vi "Main.vi"(7 "sweep rate, /min":dbl=0.2, 8 "sweep to:":dbl=-0.5, 9 "sweep":T3(radio)=enum."time_sweep") -> ()   [LabVIEW 2017] (continued)
                          frame #12 {
                            # "check if voltage \non 2400 SouceMeter 3\nis to be measured"
                            n778 = property on="data" class="Arr (strict)"() -> ("Value"=w931:dbl[])  [unwired: 2 in, 2 out]
                            n779 = local read "2400 3 meas v"() -> (w930:bool)
                            n780 = case shown="True" w930 {
                              tunnel: w931 -> [w933 w944]
                              tunnel: [w933 w943] -> w932
                              frame False {
                                # "we are not measuring 2400 3, voltage (2400_3_v)"
                              }
                              frame True {
                                # "we are  measuring 2400 3, voltage (2400_3_v)"
                                n781 = local read "2400 3 addr"() -> (w938:u8)
                                n782 = Number To Decimal String(number=w938) -> (decimal integer string=w937:string)  [unwired: 1 in]
                                n783 = GPIB Write(0:w937, 1:":READ?") -> (6:w942:errorcluster)  [unwired: 3 in, 1 out]
                                n784 = GPIB Read(0:w937, 1:3200, 3:w942) -> (5:w935:string)  [unwired: 2 in, 2 out]
                                n785 = String Subset(string=w935, length (rest)=13) -> (substring=w934:string)  [unwired: 1 in]
                                n786 = Fract/Exp String To Number(string=w934) -> (number=w940:dbl)  [unwired: 3 in, 1 out]
                                n787 = Build Array (concatenate)(w944, w940) -> (w943:dbl[])
                              }
                            }
                            n788 = property on="data" class="Arr (strict)"("Value"=w932) -> ()  [unwired: 2 in, 2 out]
                          }
                          frame #13 {
                            # "check if current \non 2400 SouceMeter 3\nis to be measured"
                            n789 = property on="data" class="Arr (strict)"() -> ("Value"=w946:dbl[])  [unwired: 2 in, 2 out]
                            n790 = local read "2400 3 meas i"() -> (w945:bool)
                            n791 = case shown="True" w945 {
                              tunnel: w946 -> [w948 w960]
                              tunnel: [w948 w959] -> w947
                              frame False {
                                # "we are not measuring 2400 3, current (2400_3_i)"
                              }
                              frame True {
                                # "we are  measuring 2400 3, current (2400_3_i)"
                                n792 = local read "2400 3 addr"() -> (w954:u8)
                                n793 = Number To Decimal String(number=w954) -> (decimal integer string=w953:string)  [unwired: 1 in]
                                n794 = GPIB Write(0:w953, 1:":READ?") -> (6:w958:errorcluster)  [unwired: 3 in, 1 out]
                                n795 = GPIB Read(0:w953, 1:3200, 3:w958) -> (5:w951:string)  [unwired: 2 in, 2 out]
                                n796 = String Subset(string=w951, offset (0)=14, length (rest)=13) -> (substring=w950:string)
                                n797 = Fract/Exp String To Number(string=w950) -> (number=w956:dbl)  [unwired: 3 in, 1 out]
                                n798 = Build Array (concatenate)(w960, w956) -> (w959:dbl[])
                              }
                            }
                            n799 = property on="data" class="Arr (strict)"("Value"=w947) -> ()  [unwired: 2 in, 2 out]
                          }
                          frame #14 {
                            # "check if 1st channel \non Keithley 2182A 1\nis to be measured"
                            n800 = property on="data" class="Arr (strict)"() -> ("Value"=w962:dbl[])  [unwired: 2 in, 2 out]
                            n801 = local read "2182A 1 ch1"() -> (w961:bool)
                            n802 = case shown="True" w961 {
                              tunnel: w962 -> [w964 w973]
                              tunnel: [w964 w972] -> w963
                              frame False {
                                # "we are not measuring 2182A 1 channel 1 (2182A_1_ch1)"
                              }
                              frame True {
                                # "we are  measuring 2182A 1 channel 1 (2182A_1_ch1)"
                                n803 = local read "2182A 1 addr"() -> (w967:u8)
                                n804 = Number To Decimal String(number=w967) -> (decimal integer string=w966:string)  [unwired: 1 in]
                                n805 = GPIB Write(0:w966, 1:":SENSe:DATA:FRES?") -> (6:w971:errorcluster)  [unwired: 3 in, 1 out]
                                n806 = GPIB Read(0:w966, 1:200, 3:w971) -> (5:w965:string)  [unwired: 2 in, 2 out]
                                n807 = Fract/Exp String To Number(string=w965) -> (number=w969:dbl)  [unwired: 3 in, 1 out]
                                n808 = Build Array (concatenate)(w973, w969) -> (w972:dbl[])
                              }
                            }
                            n809 = property on="data" class="Arr (strict)"("Value"=w963) -> ()  [unwired: 2 in, 2 out]
                          }
                          frame #15 {
                            # "check if 2nd channel \non Keithley 2182A 1\nis to be measured"
                            n810 = property on="data" class="Arr (strict)"() -> ("Value"=w975:dbl[])  [unwired: 2 in, 2 out]
                            n811 = local read "2182A 1 ch2"() -> (w974:bool)
                            n812 = case shown="True" w974 {
                              tunnel: w975 -> [w977 w990]
                              tunnel: [w977 w989] -> w976
                              frame False {
                                # "we are not measuring 2182A 1 channel 2 (2182A_1_ch2)"
                              }
                              frame True {
                                # "switching to channel 2 and then\nback to channel 1"
                                # "we are  measuring 2182A 1 channel 2 (2182A_1_ch2)"
                                n813 = local read "2182A 1 addr"() -> (w984:u8)
                                n814 = Number To Decimal String(number=w984) -> (decimal integer string=w979:string)  [unwired: 1 in]
                                n815 = GPIB Write(0:w979, 1:":SENSe:CHAN 2") -> (6:w981:errorcluster)  [unwired: 3 in, 1 out]
                                n816 = GPIB Write(0:w979, 1:":SENSe:DATA:FRES?", 3:w981) -> (6:w988:errorcluster)  [unwired: 2 in, 1 out]
                                n817 = GPIB Read(0:w979, 1:200, 3:w988) -> (5:w983:string, 7:w980:errorcluster)  [unwired: 2 in, 1 out]
                                n818 = GPIB Write(0:w979, 1:":SENSe:CHAN 1", 3:w980) -> ()  [unwired: 2 in, 2 out]
                                n819 = Fract/Exp String To Number(string=w983) -> (number=w986:dbl)  [unwired: 3 in, 1 out]
                                n820 = Build Array (concatenate)(w990, w986) -> (w989:dbl[])
                              }
                            }
                            n821 = property on="data" class="Arr (strict)"("Value"=w976) -> ()  [unwired: 2 in, 2 out]
                          }
                          frame #16 {
                            # "check if 1st channel \non Keithley 2182A 2\nis to be measured"
                            n822 = property on="data" class="Arr (strict)"() -> ("Value"=w992:dbl[])  [unwired: 2 in, 2 out]
                            n823 = local read "2182A 2 ch1"() -> (w991:bool)
                            n824 = case shown="False" w991 {
                              tunnel: w992 -> [w994 w1003]
                              tunnel: [w994 w1002] -> w993
                              frame False {
                                # "we are not measuring 2182A 2 channel 1 (2182A_2_ch1)"
                              }
                              frame True {
                                # "we are  measuring 2182A 2 channel 1 (2182A_2_ch1)"
                                n825 = local read "2182A 2 addr"() -> (w997:u8)
                                n826 = Number To Decimal String(number=w997) -> (decimal integer string=w996:string)  [unwired: 1 in]
                                n827 = GPIB Write(0:w996, 1:":SENSe:DATA:FRES?") -> (6:w1001:errorcluster)  [unwired: 3 in, 1 out]
                                n828 = GPIB Read(0:w996, 1:200, 3:w1001) -> (5:w995:string)  [unwired: 2 in, 2 out]
                                n829 = Fract/Exp String To Number(string=w995) -> (number=w999:dbl)  [unwired: 3 in, 1 out]
                                n830 = Build Array (concatenate)(w1003, w999) -> (w1002:dbl[])
                              }
                            }
                            n831 = property on="data" class="Arr (strict)"("Value"=w993) -> ()  [unwired: 2 in, 2 out]
                          }
                          frame #17 {
                            # "check if 2nd channel \non Keithley 2182A 2\nis to be measured"
                            n832 = property on="data" class="Arr (strict)"() -> ("Value"=w1005:dbl[])  [unwired: 2 in, 2 out]
                            n833 = local read "2182A 2 ch2"() -> (w1004:bool)
                            n834 = case shown="True" w1004 {
                              tunnel: w1005 -> [w1007 w1020]
                              tunnel: [w1007 w1019] -> w1006
                              frame False {
                                # "we are not measuring 2182A 2 channel 2 (2182A_2_ch2)"
                              }
                              frame True {
                                # "switching to channel 2 and then\nback to channel 1"
                                # "we are  measuring 2182A 2 channel 2 (2182A_2_ch2)"
                                n835 = local read "2182A 2 addr"() -> (w1014:u8)
                                n836 = Number To Decimal String(number=w1014) -> (decimal integer string=w1009:string)  [unwired: 1 in]
                                n837 = GPIB Write(0:w1009, 1:":SENSe:CHAN 2") -> (6:w1011:errorcluster)  [unwired: 3 in, 1 out]
                                n838 = GPIB Write(0:w1009, 1:":SENSe:DATA:FRES?", 3:w1011) -> (6:w1018:errorcluster)  [unwired: 2 in, 1 out]
                                n839 = GPIB Read(0:w1009, 1:200, 3:w1018) -> (5:w1013:string, 7:w1010:errorcluster)  [unwired: 2 in, 1 out]
                                n840 = GPIB Write(0:w1009, 1:":SENSe:CHAN 1", 3:w1010) -> ()  [unwired: 2 in, 2 out]
                                n841 = Fract/Exp String To Number(string=w1013) -> (number=w1016:dbl)  [unwired: 3 in, 1 out]
                                n842 = Build Array (concatenate)(w1020, w1016) -> (w1019:dbl[])
                              }
                            }
                            n843 = property on="data" class="Arr (strict)"("Value"=w1006) -> ()  [unwired: 2 in, 2 out]
                          }
                          frame #18 {
                            # "check if 1st channel \non Keithley 2182A 3\nis to be measured"
                            n844 = property on="data" class="Arr (strict)"() -> ("Value"=w1022:dbl[])  [unwired: 2 in, 2 out]
                            n845 = local read "2182A 3 ch1"() -> (w1021:bool)
                            n846 = case shown="True" w1021 {
                              tunnel: w1022 -> [w1024 w1033]
                              tunnel: [w1024 w1032] -> w1023
                              frame False {
                                # "we are not measuring 2182A 3 channel 1 (2182A_3_ch1)"
                              }
                              frame True {
                                # "we are  measuring 2182A 3 channel 1 (2182A_3_ch1)"
                                n847 = local read "2182A 3 addr"() -> (w1027:u8)
                                n848 = Number To Decimal String(number=w1027) -> (decimal integer string=w1026:string)  [unwired: 1 in]
                                n849 = GPIB Write(0:w1026, 1:":SENSe:DATA:FRES?") -> (6:w1031:errorcluster)  [unwired: 3 in, 1 out]
                                n850 = GPIB Read(0:w1026, 1:200, 3:w1031) -> (5:w1025:string)  [unwired: 2 in, 2 out]
                                n851 = Fract/Exp String To Number(string=w1025) -> (number=w1029:dbl)  [unwired: 3 in, 1 out]
                                n852 = Build Array (concatenate)(w1033, w1029) -> (w1032:dbl[])
                              }
                            }
                            n853 = property on="data" class="Arr (strict)"("Value"=w1023) -> ()  [unwired: 2 in, 2 out]
                          }
                          frame #19 {
                            # "check if 2nd channel \non Keithley 2182A 3\nis to be measured"
                            n854 = property on="data" class="Arr (strict)"() -> ("Value"=w1035:dbl[])  [unwired: 2 in, 2 out]
                            n855 = local read "2182A 3 ch2"() -> (w1034:bool)
                            n856 = case shown="True" w1034 {
                              tunnel: w1035 -> [w1037 w1050]
                              tunnel: [w1037 w1049] -> w1036
                              frame False {
                                # "we are not measuring 2182A 3 channel 2 (2182A_3_ch2)"
                              }
                              frame True {
                                # "switching to channel 2 and then\nback to channel 1"
                                # "we are  measuring 2182A 3 channel 2 (2182A_3_ch2)"
                                n857 = local read "2182A 3 addr"() -> (w1044:u8)
                                n858 = Number To Decimal String(number=w1044) -> (decimal integer string=w1039:string)  [unwired: 1 in]
                                n859 = GPIB Write(0:w1039, 1:":SENSe:CHAN 2") -> (6:w1041:errorcluster)  [unwired: 3 in, 1 out]
                                n860 = GPIB Write(0:w1039, 1:":SENSe:DATA:FRES?", 3:w1041) -> (6:w1048:errorcluster)  [unwired: 2 in, 1 out]
                                n861 = GPIB Read(0:w1039, 1:200, 3:w1048) -> (5:w1043:string, 7:w1040:errorcluster)  [unwired: 2 in, 1 out]
                                n862 = GPIB Write(0:w1039, 1:":SENSe:CHAN 1", 3:w1040) -> ()  [unwired: 2 in, 2 out]
                                n863 = Fract/Exp String To Number(string=w1043) -> (number=w1046:dbl)  [unwired: 3 in, 1 out]
                                n864 = Build Array (concatenate)(w1050, w1046) -> (w1049:dbl[])
                              }
                            }
                            n865 = property on="data" class="Arr (strict)"("Value"=w1036) -> ()  [unwired: 2 in, 2 out]
                          }
                          frame #20 {
                            # "check if 1st channel \non Keithley 2182A 4\nis to be measured"
                            n866 = property on="data" class="Arr (strict)"() -> ("Value"=w1052:dbl[])  [unwired: 2 in, 2 out]
                            n867 = local read "2182A 4 ch1"() -> (w1051:bool)
                            n868 = case shown="True" w1051 {
                              tunnel: w1052 -> [w1054 w1063]
                              tunnel: [w1054 w1062] -> w1053
                              frame False {
                                # "we are not measuring 2182A 4 channel 1 (2182A_4_ch1)"
                              }
                              frame True {
                                # "we are  measuring 2182A 4 channel 1 (2182A_4_ch1)"
                                n869 = local read "2182A 4 addr"() -> (w1057:u8)
                                n870 = Number To Decimal String(number=w1057) -> (decimal integer string=w1056:string)  [unwired: 1 in]
                                n871 = GPIB Write(0:w1056, 1:":SENSe:DATA:FRES?") -> (6:w1061:errorcluster)  [unwired: 3 in, 1 out]
                                n872 = GPIB Read(0:w1056, 1:200, 3:w1061) -> (5:w1055:string)  [unwired: 2 in, 2 out]
                                n873 = Fract/Exp String To Number(string=w1055) -> (number=w1059:dbl)  [unwired: 3 in, 1 out]
                                n874 = Build Array (concatenate)(w1063, w1059) -> (w1062:dbl[])
                              }
                            }
                            n875 = property on="data" class="Arr (strict)"("Value"=w1053) -> ()  [unwired: 2 in, 2 out]
                          }
                          frame #21 {
                            # "check if 2nd channel \non Keithley 2182A 4\nis to be measured"
                            n876 = property on="data" class="Arr (strict)"() -> ("Value"=w1065:dbl[])  [unwired: 2 in, 2 out]
                            n877 = local read "2182A 4 ch2"() -> (w1064:bool)
                            n878 = case shown="False" w1064 {
                              tunnel: w1065 -> [w1067 w1080]
                              tunnel: [w1067 w1079] -> w1066
                              frame False {
                                # "we are not measuring 2182A 4 channel 2 (2182A_4_ch2)"
                              }
                              frame True {
                                # "switching to channel 2 and then\nback to channel 1"
                                # "we are  measuring 2182A 4 channel 2 (2182A_4_ch2)"
                                n879 = local read "2182A 4 addr"() -> (w1074:u8)
                                n880 = Number To Decimal String(number=w1074) -> (decimal integer string=w1069:string)  [unwired: 1 in]
                                n881 = GPIB Write(0:w1069, 1:":SENSe:CHAN 2") -> (6:w1071:errorcluster)  [unwired: 3 in, 1 out]
                                n882 = GPIB Write(0:w1069, 1:":SENSe:DATA:FRES?", 3:w1071) -> (6:w1078:errorcluster)  [unwired: 2 in, 1 out]
                                n883 = GPIB Read(0:w1069, 1:200, 3:w1078) -> (5:w1073:string, 7:w1070:errorcluster)  [unwired: 2 in, 1 out]
                                n884 = GPIB Write(0:w1069, 1:":SENSe:CHAN 1", 3:w1070) -> ()  [unwired: 2 in, 2 out]
                                n885 = Fract/Exp String To Number(string=w1073) -> (number=w1076:dbl)  [unwired: 3 in, 1 out]
                                n886 = Build Array (concatenate)(w1080, w1076) -> (w1079:dbl[])
                              }
                            }
                            n887 = property on="data" class="Arr (strict)"("Value"=w1066) -> ()  [unwired: 2 in, 2 out]
                          }
                          frame #22 {
                            # "check if voltage on\nKeithley 2636A smua\nis to be measured"
                            n888 = local read "2636A smua meas v"() -> (w1081:bool)
                            n889 = property on="data" class="Arr (strict)"() -> ("Value"=w1082:dbl[])  [unwired: 2 in, 2 out]
                            n890 = case shown="True" w1081 {
                              tunnel: w1082 -> [w1084 w1090]
                              tunnel: [w1084 w1089] -> w1083
                              frame False {
                                # "we are not measuring voltage on 2636A smua (2636A_smua_v)"
                              }
                              frame True {
                                # "we are  measuring voltage on 2636A smua (2636A_smua_v)"
                                n891 = local read "2336A addr"() -> (w1085:refnum<visa-resource-name>)
                                n892 = call "SinglePointMeasurement.vi"("Measure"=Measure."Voltage", "Channel"=Channel."a", "VISA resource name 2"=w1085) -> ("Measuremet"=w1087:dbl)  [unwired: 3 in, 4 out]
                                n893 = Build Array (concatenate)(w1090, w1087) -> (w1089:dbl[])
                              }
                            }
                            n894 = property on="data" class="Arr (strict)"("Value"=w1083) -> ()  [unwired: 2 in, 2 out]
                          }
                          frame #23 {
                            # "check if current on\nKeithley 2636A smua\nis to be measured"
                            n895 = local read "2636A smua meas i"() -> (w1091:bool)
                            n896 = property on="data" class="Arr (strict)"() -> ("Value"=w1092:dbl[])  [unwired: 2 in, 2 out]
                            n897 = case shown="True" w1091 {
                              tunnel: w1092 -> [w1094 w1097]
                              tunnel: [w1094 w1096] -> w1093
                              frame False {
                                # "we are not measuring current on 2636A smua (2636A_smua_i)"
                              }
                              frame True {
                                # "we are  measuring current on 2636A smua (2636A_smua_i)"
                                n898 = stacked-sequence {
                                tunnel: [_ w1106] -> w1095
                                frame #0 {
                                n899 = local read "auto\nrange A"() -> (w1101:bool)
                                n900 = local read "2336A addr"() -> (w1104:refnum<visa-resource-name>)
                                n901 = Select(t="smua.AUTORANGE_ON", s=w1101, f="smua.AUTORANGE_OFF") -> (s? t:f=w1099:string)
                                n902 = Concatenate Strings("smua.measure.autorangei = ", w1099) -> (w1098:string)
                                n903 = VISA Write(VISA resource name=w1104, write buffer=w1098) -> ()  [unwired: 1 in, 3 out]
                                }
                                frame #1 {
                                n904 = local read "2336A addr"() -> (w1108:refnum<visa-resource-name>)
                                n905 = call "SinglePointMeasurement.vi"("Measure"=Measure."Current", "Channel"=Channel."a", "VISA resource name 2"=w1108) -> ("Measuremet"=w1106:dbl)  [unwired: 3 in, 4 out]
                                }
                                }
                                n906 = Build Array (concatenate)(w1097, w1095) -> (w1096:dbl[])
                              }
                            }
                            n907 = property on="data" class="Arr (strict)"("Value"=w1093) -> ()  [unwired: 2 in, 2 out]
                          }
                          frame #24 {
                            # "check if voltage on\nKeithley 2636A smub\nis to be measured"
                            n908 = local read "2636A smub meas v"() -> (w1109:bool)
                            n909 = property on="data" class="Arr (strict)"() -> ("Value"=w1110:dbl[])  [unwired: 2 in, 2 out]
                            n910 = case shown="True" w1109 {
                              tunnel: w1110 -> [w1112 w1118]
                              tunnel: [w1112 w1117] -> w1111
                              frame False {
                                # "we are not measuring voltage on 2636A smub (2636A_smub_v)"
                              }
                              frame True {
                                # "we are  measuring voltage on 2636A smub (2636A_smub_v)"
                                n911 = local read "2336A addr"() -> (w1116:refnum<visa-resource-name>)
                                n912 = call "SinglePointMeasurement.vi"("Measure"=Measure."Voltage", "Channel"=Channel."b", "VISA resource name 2"=w1116) -> ("Measuremet"=w1114:dbl)  [unwired: 3 in, 4 out]
                                n913 = Build Array (concatenate)(w1118, w1114) -> (w1117:dbl[])
                              }
                            }
                            n914 = property on="data" class="Arr (strict)"("Value"=w1111) -> ()  [unwired: 2 in, 2 out]
                          }
                          frame #25 {
                            # "check if current on\nKeithley 2636A smub\nis to be measured"
                            n915 = local read "2636A smub meas i"() -> (w1119:bool)
                            n916 = property on="data" class="Arr (strict)"() -> ("Value"=w1120:dbl[])  [unwired: 2 in, 2 out]
                            n917 = case shown="True" w1119 {
                              tunnel: w1120 -> [w1122 w1125]
                              tunnel: [w1122 w1124] -> w1121
                              frame False {
                                # "we are not measuring current on 2636A smub (2636A_smub_i)"
                              }
                              frame True {
                                # "we are  measuring current on 2636A smub (2636A_smub_i)"
                                n918 = stacked-sequence {
                                tunnel: [_ w1134] -> w1123
                                frame #0 {
                                n919 = local read "auto\nrange B"() -> (w1129:bool)
                                n920 = local read "2336A addr"() -> (w1132:refnum<visa-resource-name>)
                                n921 = Select(t="smub.AUTORANGE_ON", s=w1129, f="smub.AUTORANGE_OFF") -> (s? t:f=w1127:string)
                                n922 = Concatenate Strings("smub.measure.autorangei = ", w1127) -> (w1126:string)
                                n923 = VISA Write(VISA resource name=w1132, write buffer=w1126) -> ()  [unwired: 1 in, 3 out]
                                }
                                frame #1 {
                                n924 = local read "2336A addr"() -> (w1136:refnum<visa-resource-name>)
                                n925 = call "SinglePointMeasurement.vi"("Measure"=Measure."Current", "Channel"=Channel."b", "VISA resource name 2"=w1136) -> ("Measuremet"=w1134:dbl)  [unwired: 3 in, 4 out]
                                }
                                }
                                n926 = Build Array (concatenate)(w1125, w1123) -> (w1124:dbl[])
                              }
                            }
                            n927 = property on="data" class="Arr (strict)"("Value"=w1121) -> ()  [unwired: 2 in, 2 out]
                          }
                          frame #26 {
                            # "check if time\nis to be measured"
                            n928 = property on="data" class="Arr (strict)"() -> ("Value"=w1138:dbl[])  [unwired: 2 in, 2 out]
                            n929 = local read "measure time"() -> (w1137:bool)
                            n930 = case shown="True" w1137 {
                              tunnel: w1138 -> [w1140 w1143]
                              tunnel: [w1140 w1142] -> w1139
                              frame False {
                                # "we are not measuring time"
                              }
                              frame True {
                                # "seconds from the beginning of month"
                                # "we are  measuring time"
                                n931 = Build Array (concatenate)(w1143, 0) -> (w1142:dbl[])
                              }
                            }
                            n932 = property on="data" class="Arr (strict)"("Value"=w1139) -> ()  [unwired: 2 in, 2 out]
                          }
                          frame #27 {
                            n933 = local read "iPS_MagnetField"() -> (w1145:bool)
                            n934 = property on="data" class="Arr (strict)"() -> ("Value"=w1146:dbl[])  [unwired: 2 in, 2 out]
                            n935 = case shown="True" w1145 {
                              tunnel: w1146 -> [_ w1155]
                              tunnel: [_ w1154] -> w1144
                              frame False {
                                # "we are not Measuring magnetic field on IPS120-0"
                              }
                              frame True {
                                w1149 = 1
                                # "Measure magnetic field on IPS120-0"
                                n936 = local read "IPS120-0 addr_sweep"() -> (w1151:u8)
                                n937 = Number To Decimal String(number=w1151) -> (decimal integer string=w1152:string)  [unwired: 1 in]
                                n938 = GPIB Write(0:w1152, 1:"R 7", 2:w1149) -> ()  [unwired: 2 in, 2 out]
                                n939 = GPIB Read(0:w1152, 1:200 ("byte count"), 2:w1149) -> (5:w1153:string)  [unwired: 2 in, 2 out]
                                n940 = Fract/Exp String To Number(string=w1153, offset=w1149) -> (number=w1147:dbl)  [unwired: 2 in, 1 out]
                                n941 = Build Array (concatenate)(w1155, w1147) -> (w1154:dbl[])
                              }
                            }
                            n942 = property on="data" class="Arr (strict)"("Value"=w1144) -> ()  [unwired: 2 in, 2 out]
                          }
                          frame #28 {
                            # "check if current \non 2461 SouceMeter\nis to be measured"
                            n943 = property on="data" class="Arr (strict)"() -> ("Value"=w1158:dbl[])  [unwired: 2 in, 2 out]
                            n944 = property on="iTC_Sample_T" class="Bool (strict)"() -> ("Value"=w1157:bool)  [unwired: 2 in, 2 out]
                            n945 = case shown="True" w1157 {
                              tunnel: w1158 -> [_ w1171]
                              tunnel: [_ w1170] -> w1156
                              frame False {
                                # "we are not measuring 2461, voltage (2461_meas_v)"
                              }
                              frame True {
                                w1160 = 1
                                # "temporarily ITC503S"
                                # "we are  measuring  Teslatron_iTC_Temp"
                                n946 = property on="iTC_503_addr_sweep" class="DigNum (strict)"() -> ("Value"=w1165:u8)  [unwired: 2 in, 2 out]
                                n947 = Number To Decimal String(number=w1165) -> (decimal integer string=w1166:string)  [unwired: 1 in]
                                n948 = GPIB Write(0:w1166, 1:"$C3", 2:1) -> (6:w1167:errorcluster)  [unwired: 2 in, 1 out]
                                n949 = GPIB Write(0:w1166, 1:"R3", 2:w1160, 3:w1167) -> (6:w1169:errorcluster)  [unwired: 1 in, 1 out]
                                n950 = GPIB Read(0:w1166, 1:200, 2:w1160, 3:w1169) -> (5:w1168:string)  [unwired: 1 in, 2 out]
                                n951 = Fract/Exp String To Number(string=w1168, offset=w1160) -> (number=w1159:dbl)  [unwired: 2 in, 1 out]
                                n952 = Build Array (concatenate)(w1171, w1159) -> (w1170:dbl[])
                              }
                            }
                            n953 = property on="data" class="Arr (strict)"("Value"=w1156) -> ()  [unwired: 2 in, 2 out]
                          }
                          frame #29 {
                            # "check if current \non 2461 SouceMeter\nis to be measured"
                            n954 = property on="CH_A" class="Bool (strict)"() -> ("Value"=w1172:bool)  [unwired: 2 in, 2 out]
                            n955 = property on="data" class="Arr (strict)"() -> ("Value"=w1173:dbl[])  [unwired: 2 in, 2 out]
                            n956 = case shown="True" w1172 {
                              tunnel: w1173 -> [w1175 w1188]
                              tunnel: [w1175 w1187] -> w1174
                              frame False {
                                # "we are not measuring 2461, voltage (2461_meas_v)"
                              }
                              frame True {
                                w1180 = 1
                                # "temporarily ITC503S"
                                # "we are  measuring  Teslatron_iTC_Temp"
                                n957 = property on="iTC_503_addr_sweep" class="DigNum (strict)"() -> ("Value"=w1182:u8)  [unwired: 2 in, 2 out]
                                n958 = Number To Decimal String(number=w1182) -> (decimal integer string=w1183:string)  [unwired: 1 in]
                                n959 = GPIB Write(0:w1183, 1:"$C3", 2:1) -> (6:w1184:errorcluster)  [unwired: 2 in, 1 out]
                                n960 = GPIB Write(0:w1183, 1:"R3", 2:w1180, 3:w1184) -> (6:w1186:errorcluster)  [unwired: 1 in, 1 out]
                                n961 = GPIB Read(0:w1183, 1:200, 2:w1180, 3:w1186) -> (5:w1185:string)  [unwired: 1 in, 2 out]
                                n962 = Fract/Exp String To Number(string=w1185, offset=w1180) -> (number=w1181:dbl)  [unwired: 2 in, 1 out]
                                n963 = Build Array (concatenate)(w1188, w1181) -> (w1187:dbl[])
                              }
                            }
                            n964 = property on="data" class="Arr (strict)"("Value"=w1174) -> ()  [unwired: 2 in, 2 out]
                          }
                          frame #30 {
                            # "check if current \non 2461 SouceMeter\nis to be measured"
                            n965 = property on="CH_B" class="Bool (strict)"() -> ("Value"=w1189:bool)  [unwired: 2 in, 2 out]
                            n966 = property on="data" class="Arr (strict)"() -> ("Value"=w1190:dbl[])  [unwired: 2 in, 2 out]
                            n967 = case shown="True" w1189 {
                              tunnel: w1190 -> [w1192 w1205]
                              tunnel: [w1192 w1204] -> w1191
                              frame False {
                                # "we are not measuring 2461, voltage (2461_meas_v)"
                              }
                              frame True {
                                w1196 = 1
                                # "temporarily ITC503S"
                                # "we are  measuring  Teslatron_iTC_Temp"
                                n968 = property on="iTC_503_addr_sweep" class="DigNum (strict)"() -> ("Value"=w1199:u8)  [unwired: 2 in, 2 out]
                                n969 = Number To Decimal String(number=w1199) -> (decimal integer string=w1200:string)  [unwired: 1 in]
                                n970 = GPIB Write(0:w1200, 1:"$C3", 2:1) -> (6:w1201:errorcluster)  [unwired: 2 in, 1 out]
                                n971 = GPIB Write(0:w1200, 1:"R2", 2:w1196, 3:w1201) -> (6:w1203:errorcluster)  [unwired: 1 in, 1 out]
                                n972 = GPIB Read(0:w1200, 1:200, 2:w1196, 3:w1203) -> (5:w1202:string)  [unwired: 1 in, 2 out]
                                n973 = Fract/Exp String To Number(string=w1202, offset=w1196) -> (number=w1193:dbl)  [unwired: 2 in, 1 out]
                                n974 = Build Array (concatenate)(w1205, w1193) -> (w1204:dbl[])
                              }
                            }
                            n975 = property on="data" class="Arr (strict)"("Value"=w1191) -> ()  [unwired: 2 in, 2 out]
                          }
                        }
                      }
                    }
                  }
                }
              }
            }
          }
          frame #3 {
            n976 = Enqueue Element(queue=w1206, element="Idle") -> ()  [unwired: 2 in, 3 out]
            n977 = Wait (ms)(milliseconds to wait="Refresh Time(ms)") -> ()  [unwired: 1 out]
          }
        }
      }
      frame "Start Sweep" {
        w1212 = dbl[][] []  # emty array for data
        # "0 = SR830_1_ip\n1 = SR830_1_oop\n2 = SR830_2_ip\n3 = SR830_2_oop\n4 = SR830_3_ip\n5 = SR830_3_oop\n6 = SR830_4_ip \n7 = SR830_4_oop \n8= 2400_1_v \n9 = 2400_1_i \n10 = 2400_2_v\n11 = 2400_2_i \n12 = 2400_3_v \n13 = 2400_3_i \n14 = 2182A_1_ch1 \n15 = 2182A_1_ch2 \n16 = 2182A_2_ch1 \n17 = 2182A_2_ch2\n18 = 2182A_3_ch1 \n19 = 2182A_3_ch2 \n20 = 2182A_4_ch1 \n21 = 2182A_4_ch2 \n22 = 2636A_smua_v \n23 = 2636A_smua_i \n24 = 2636A_smub_v \n25 = 2636A_smub_i \n26 = time\n27 = iPS_120\n28 = iTC _sample_T\n28 = iTC _CH_A\n29=iTC_CH_B\n31 = Step_Value"
        # "initial time in seconds\nfrom the beginning of month"
        n978 = call "timeInSeconds.vi"() -> ("Numeric"=w1213:dbl)  [unwired: 2 in, 1 out]
        n979 = stacked-sequence {
          tunnel: [_ _ w1755 _ _ _] -> w1209
          frame #0 {
            n980 = local read "2636A smua meas v"() -> (w1219:bool)
            n981 = local read "2636A smub meas v"() -> (w1217:bool)
            n982 = local read "2636A smub meas i"() -> (w1216:bool)
            n983 = local read "2636A smua meas i"() -> (w1218:bool)
            n984 = property on="sweep" class="RadioBtnsControl (strict)"() -> ("Value"=w1214:T3)  [unwired: 2 in, 2 out]
            n985 = Compound Arithmetic op=OR(w1219, w1218, w1217, w1216) -> (w1215:bool)
            n986 = case shown="\"2400_3\"" w1214 {
              frame "2400_1" {
                # "add label for the first column in the datafile"
                n987 = stacked-sequence {
                  frame #0 {
                    n988 = property on="data_caption" class="Str"("Value"="") -> ()  [unwired: 2 in, 2 out]
                    n989 = property on="Figure_axis" class="Arr (strict)"("Value"=string[] [] ("Figure_axis_string")) -> ()  [unwired: 2 in, 2 out]
                  }
                  frame #1 {
                    w1222 = "V_sweep_2400_1" ("V_sweep")
                    n990 = Concatenate Strings(w1222, "\t") -> (w1224:string)
                    n991 = Build Array(w1222) -> (w1223:string[])
                    n992 = property on="data_caption" class="Str"("Value"=w1224) -> ()  [unwired: 2 in, 2 out]
                    n993 = property on="Figure_axis" class="Arr (strict)"("Value"=w1223) -> ()  [unwired: 2 in, 2 out]
                  }
                }
              }
              frame "2400_2" {
                n994 = stacked-sequence {
                  frame #0 {
                    n995 = property on="data_caption" class="Str"("Value"="") -> ()  [unwired: 2 in, 2 out]
                    n996 = property on="Figure_axis" class="Arr (strict)"("Value"=string[] [] ("Figure_axis_string")) -> ()  [unwired: 2 in, 2 out]
                  }
                  frame #1 {
                    w1228 = "V_sweep_2400_2" ("V_sweep")
                    n997 = Build Array(w1228) -> (w1229:string[])
                    n998 = Concatenate Strings(w1228, "\t") -> (w1231:string)
                    n999 = property on="Figure_axis" class="Arr (strict)"("Value"=w1229) -> ()  [unwired: 2 in, 2 out]
                    n1000 = property on="data_caption" class="Str"("Value"=w1231) -> ()  [unwired: 2 in, 2 out]
                  }
                }
              }
              frame "2400_3" {
                n1001 = stacked-sequence {
                  frame #0 {
                    n1002 = property on="data_caption" class="Str"("Value"="") -> ()  [unwired: 2 in, 2 out]
                    n1003 = property on="Figure_axis" class="Arr (strict)"("Value"=string[] [] ("Figure_axis_string")) -> ()  [unwired: 2 in, 2 out]
                  }
                  frame #1 {
                    w1234 = "V_sweep_2400_3" ("V_sweep")
                    n1004 = Concatenate Strings(w1234, "\t") -> (w1237:string)
                    n1005 = Build Array(w1234) -> (w1235:string[])
                    n1006 = property on="data_caption" class="Str"("Value"=w1237) -> ()  [unwired: 2 in, 2 out]
                    n1007 = property on="Figure_axis" class="Arr (strict)"("Value"=w1235) -> ()  [unwired: 2 in, 2 out]
                  }
                }
              }
              frame "2636a_smua" {
                n1008 = stacked-sequence {
                  frame #0 {
                    n1009 = property on="data_caption" class="Str"("Value"="") -> ()  [unwired: 2 in, 2 out]
                    n1010 = property on="Figure_axis" class="Arr (strict)"("Value"=string[] [] ("Figure_axis_string")) -> ()  [unwired: 2 in, 2 out]
                  }
                  frame #1 {
                    w1240 = "V_sweep_2636a_smua" ("V_sweep")
                    n1011 = Concatenate Strings(w1240, "\t") -> (w1243:string)
                    n1012 = Build Array(w1240) -> (w1241:string[])
                    n1013 = property on="data_caption" class="Str"("Value"=w1243) -> ()  [unwired: 2 in, 2 out]
                    n1014 = property on="Figure_axis" class="Arr (strict)"("Value"=w1241) -> ()  [unwired: 2 in, 2 out]
                  }
                }
              }
              frame "2636a_smub" {
                n1015 = stacked-sequence {
                  frame #0 {
                    n1016 = property on="data_caption" class="Str"("Value"="") -> ()  [unwired: 2 in, 2 out]
                    n1017 = property on="Figure_axis" class="Arr (strict)"("Value"=string[] [] ("Figure_axis_string")) -> ()  [unwired: 2 in, 2 out]
                  }
                  frame #1 {
                    w1246 = "V_sweep_2636a_smub" ("V_sweep")
                    n1018 = Build Array(w1246) -> (w1247:string[])
                    n1019 = Concatenate Strings(w1246, "\t") -> (w1249:string)
                    n1020 = property on="Figure_axis" class="Arr (strict)"("Value"=w1247) -> ()  [unwired: 2 in, 2 out]
                    n1021 = property on="data_caption" class="Str"("Value"=w1249) -> ()  [unwired: 2 in, 2 out]
                  }
                }
              }
              frame "time_sweep", Default {
                n1022 = stacked-sequence {
                  frame #0 {
                    n1023 = property on="data_caption" class="Str"("Value"="") -> ()  [unwired: 2 in, 2 out]
                    n1024 = property on="Figure_axis" class="Arr (strict)"("Value"=string[] [] ("Figure_axis_string")) -> ()  [unwired: 2 in, 2 out]
                  }
                  frame #1 {
                    w1252 = "time_sweep" ("V_sweep")
                    n1025 = Build Array(w1252) -> (w1253:string[])
                    n1026 = Concatenate Strings(w1252, "\t") -> (w1254:string)
                    n1027 = property on="Figure_axis" class="Arr (strict)"("Value"=w1253) -> ()  [unwired: 2 in, 2 out]
                    n1028 = property on="data_caption" class="Str"("Value"=w1254) -> ()  [unwired: 2 in, 2 out]
                  }
                }
              }
              frame "iPS" {
                n1029 = stacked-sequence {
                  frame #0 {
                    n1030 = property on="data_caption" class="Str"("Value"="") -> ()  [unwired: 2 in, 2 out]
                    n1031 = property on="Figure_axis" class="Arr (strict)"("Value"=string[] [] ("Figure_axis_string")) -> ()  [unwired: 2 in, 2 out]
                  }
                  frame #1 {
                    w1258 = "Teslatron_iPS_OutputField" ("V_sweep")
                    n1032 = Build Array(w1258) -> (w1259:string[])
                    n1033 = Concatenate Strings(w1258, "\t") -> (w1261:string)
                    n1034 = property on="Figure_axis" class="Arr (strict)"("Value"=w1259) -> ()  [unwired: 2 in, 2 out]
                    n1035 = property on="data_caption" class="Str"("Value"=w1261) -> ()  [unwired: 2 in, 2 out]
                  }
                }
              }
              frame "iTC" {
                n1036 = stacked-sequence {
                  frame #0 {
                    n1037 = property on="data_caption" class="Str"("Value"="") -> ()  [unwired: 2 in, 2 out]
                    n1038 = property on="Figure_axis" class="Arr (strict)"("Value"=string[] ["", "SR830_1_ip", "SR830_1_oop", "SR830_2_ip", "SR830_2_oop", "2461_meas_v", "2461_meas_i", "2636A_smua_v", "2636A_smua_i", "formula"] ("Figure_axis")) -> ()  [unwired: 2 in, 2 out]
                  }
                  frame #1 {
                    w1266 = "Teslatron_iTC_Temp"
                    n1039 = Build Array(w1266) -> (w1265:string[])
                    n1040 = Concatenate Strings(w1266, "\t") -> (w1264:string)
                    n1041 = property on="data_caption" class="Str"("Value"=w1264) -> ()  [unwired: 2 in, 2 out]
                    n1042 = property on="Figure_axis" class="Arr (strict)"("Value"=w1265) -> ()  [unwired: 2 in, 2 out]
                  }
                }
              }
            }
            n1043 = case shown="True" w1215 {
              frame False {
              }
              frame True {
                # "opens session for 2636a system sourcemeter"
                n1044 = local read "2336A addr"() -> (w1268:refnum<visa-resource-name>)
                n1045 = VISA Open(VISA resource name=w1268) -> ()  [unwired: 4 in, 2 out]
              }
            }
          }
          frame #1 {
            # "0 = SR830_1_ip\n1 = SR830_1_oop\n2 = SR830_2_ip\n3 = SR830_2_oop\n4 = SR830_3_ip\n5 = SR830_3_oop\n6 = SR830_4_ip \n7 = SR830_4_oop \n8= 2400_1_v \n9 = 2400_1_i \n10 = 2400_2_v\n11 = 2400_2_i \n12 = 2400_3_v \n13 = 2400_3_i \n14 = 2182A_1_ch1 \n15 = 2182A_1_ch2 \n16 = 2182A_2_ch1 \n17 = 2182A_2_ch2\n18 = 2182A_3_ch1 \n19 = 2182A_3_ch2 \n20 = 2182A_4_ch1 \n21 = 2182A_4_ch2 \n22 = 2636A_smua_v \n23 = 2636A_smua_i \n24 = 2636A_smub_v \n25 = 2636A_smub_i \n26 = time\n27 = iPS_120\n28 = iTC _sample_T\n28 = iTC _CH_A\n29=iTC_CH_B\n31 = Step_Value"
            # "this part constructs the first (text) line for the data file with names of all measured variables,\nalso constructs a text array contaning names of all measured variable for the \"ring\" (so parameter can be selected and plotted)"
            n1046 = stacked-sequence {
              tunnel: [w1269 _ _ _ _ _ _ _ _ _ _ _ _ _ _ _ _ _ _ _ _ _ _ _ _ _ _ _ _ _ _ _] -> _
              frame #0 {
                # "SR830 1 in phase (SR830_1_ip)"
                n1047 = local read "SR830 1 ip"() -> (w1274:bool)
                n1048 = property on="Figure_axis" class="Arr (strict)"() -> ("Value"=w1271:string[])  [unwired: 2 in, 2 out]
                n1049 = property on="data_caption" class="Str"() -> ("Value"=w1273:string)  [unwired: 2 in, 2 out]
                n1050 = case shown="True" w1274 {
                  tunnel: w1273 -> [w1276 w1282]
                  tunnel: [w1276 w1281] -> w1272
                  tunnel: w1271 -> [w1275 w1279]
                  tunnel: [w1275 w1277] -> w1270
                  frame False {
                    # "not measure SR830 1 in phase signal (SR830_1_ip)"
                  }
                  frame True {
                    w1278 = "SR830_1_ip"
                    # "measure SR830 1 in phase signal (SR830_1_ip)"
                    n1051 = local read "SR830 1 addr"() -> (w1283:u8)
                    n1052 = Number To Decimal String(number=w1283) -> (decimal integer string=w1284:string)  [unwired: 1 in]
                    n1053 = GPIB Clear(3:w1284) -> ()  [unwired: 1 in, 2 out]
                    n1054 = Build Array (concatenate)(w1279, w1278) -> (w1277:string[])
                    n1055 = Concatenate Strings(w1282, w1278, "\t") -> (w1281:string)
                  }
                }
                n1056 = property on="Figure_axis" class="Arr (strict)"("Value"=w1270) -> ()  [unwired: 2 in, 2 out]
                n1057 = property on="data_caption" class="Str"("Value"=w1272) -> (error out=w1269:errorcluster)  [unwired: 2 in, 1 out]
              }
              frame #1 {
                # "SR830 1 out of phase (SR830_1_oop)"
                n1058 = local read "SR830 1 oop"() -> (w1289:bool)
                n1059 = property on="Figure_axis" class="Arr (strict)"() -> ("Value"=w1286:string[])  [unwired: 2 in, 2 out]
                n1060 = property on="data_caption" class="Str"() -> ("Value"=w1288:string)  [unwired: 2 in, 2 out]
                n1061 = case shown="False" w1289 {
                  tunnel: w1288 -> [w1291 w1297]
                  tunnel: [w1291 w1296] -> w1287
                  tunnel: w1286 -> [w1290 w1294]
                  tunnel: [w1290 w1292] -> w1285
                  frame False {
                    # "not measure SR830 1 out of phase signal (SR830_1_oop)"
                  }
                  frame True {
                    w1293 = "SR830_1_oop"
                    # "measure SR830 1 out of phase signal (SR830_1_oop)"
                    n1062 = local read "SR830 1 addr"() -> (w1298:u8)
                    n1063 = Number To Decimal String(number=w1298) -> (decimal integer string=w1299:string)  [unwired: 1 in]
                    n1064 = GPIB Clear(3:w1299) -> ()  [unwired: 1 in, 2 out]
                    n1065 = Build Array (concatenate)(w1294, w1293) -> (w1292:string[])
                    n1066 = Concatenate Strings(w1297, w1293, "\t") -> (w1296:string)
                  }
                }
                n1067 = property on="Figure_axis" class="Arr (strict)"("Value"=w1285) -> ()  [unwired: 2 in, 2 out]
                n1068 = property on="data_caption" class="Str"("Value"=w1287) -> ()  [unwired: 2 in, 2 out]
              }
              frame #2 {
                # "SR830 2 in phase (SR830_2_ip)"
                n1069 = local read "SR830 2 ip"() -> (w1304:bool)
                n1070 = property on="Figure_axis" class="Arr (strict)"() -> ("Value"=w1301:string[])  [unwired: 2 in, 2 out]
                n1071 = property on="data_caption" class="Str"() -> ("Value"=w1303:string)  [unwired: 2 in, 2 out]
                n1072 = case shown="False" w1304 {
                  tunnel: w1303 -> [w1306 w1312]
                  tunnel: [w1306 w1311] -> w1302
                  tunnel: w1301 -> [w1305 w1309]
                  tunnel: [w1305 w1307] -> w1300
                  frame False {
                    # "not measure SR830 2 in phase signal (SR830_2_ip)"
                  }
                  frame True {
                    w1308 = "SR830_2_ip"
                    # "measure SR830 2 in phase signal (SR830_2_ip)"
                    n1073 = local read "SR830 2 addr"() -> (w1313:u8)
                    n1074 = Number To Decimal String(number=w1313) -> (decimal integer string=w1314:string)  [unwired: 1 in]
                    n1075 = GPIB Clear(3:w1314) -> ()  [unwired: 1 in, 2 out]
                    n1076 = Build Array (concatenate)(w1309, w1308) -> (w1307:string[])
                    n1077 = Concatenate Strings(w1312, w1308, "\t") -> (w1311:string)
                  }
                }
                n1078 = property on="Figure_axis" class="Arr (strict)"("Value"=w1300) -> ()  [unwired: 2 in, 2 out]
                n1079 = property on="data_caption" class="Str"("Value"=w1302) -> ()  [unwired: 2 in, 2 out]
              }
              frame #3 {
                # "SR830 2 out of phase (SR830_2_oop)"
                n1080 = local read "SR830 2 oop"() -> (w1319:bool)
                n1081 = property on="Figure_axis" class="Arr (strict)"() -> ("Value"=w1316:string[])  [unwired: 2 in, 2 out]
                n1082 = property on="data_caption" class="Str"() -> ("Value"=w1318:string)  [unwired: 2 in, 2 out]
                n1083 = case shown="False" w1319 {
                  tunnel: w1318 -> [w1321 w1327]
                  tunnel: [w1321 w1326] -> w1317
                  tunnel: w1316 -> [w1320 w1324]
                  tunnel: [w1320 w1322] -> w1315
                  frame False {
                    # "not measure SR830 2 out of phase signal (SR830_2_oop)"
                  }
                  frame True {
                    w1323 = "SR830_2_oop"
                    # "measure SR830 2 out of phase signal (SR830_2_oop)"
                    n1084 = local read "SR830 2 addr"() -> (w1328:u8)
                    n1085 = Number To Decimal String(number=w1328) -> (decimal integer string=w1329:string)  [unwired: 1 in]
                    n1086 = GPIB Clear(3:w1329) -> ()  [unwired: 1 in, 2 out]
                    n1087 = Build Array (concatenate)(w1324, w1323) -> (w1322:string[])
                    n1088 = Concatenate Strings(w1327, w1323, "\t") -> (w1326:string)
                  }
                }
                n1089 = property on="Figure_axis" class="Arr (strict)"("Value"=w1315) -> ()  [unwired: 2 in, 2 out]
                n1090 = property on="data_caption" class="Str"("Value"=w1317) -> ()  [unwired: 2 in, 2 out]
              }
              frame #4 {
                # "SR830 3 in phase (SR830_3_ip)"
                n1091 = local read "SR830 3 ip"() -> (w1334:bool)
                n1092 = property on="Figure_axis" class="Arr (strict)"() -> ("Value"=w1331:string[])  [unwired: 2 in, 2 out]
                n1093 = property on="data_caption" class="Str"() -> ("Value"=w1333:string)  [unwired: 2 in, 2 out]
                n1094 = case shown="False" w1334 {
                  tunnel: w1333 -> [w1336 w1342]
                  tunnel: [w1336 w1341] -> w1332
                  tunnel: w1331 -> [w1335 w1339]
                  tunnel: [w1335 w1337] -> w1330
                  frame False {
                    # "not measure SR830 3 in phase signal (SR830_3_ip)"
                  }
                  frame True {
                    w1338 = "SR830_3_ip"
                    # "measure SR830 3 in phase signal (SR830_3_ip)"
                    n1095 = local read "SR830 3 addr"() -> (w1343:u8)
                    n1096 = Number To Decimal String(number=w1343) -> (decimal integer string=w1344:string)  [unwired: 1 in]
                    n1097 = GPIB Clear(3:w1344) -> ()  [unwired: 1 in, 2 out]
                    n1098 = Build Array (concatenate)(w1339, w1338) -> (w1337:string[])
                    n1099 = Concatenate Strings(w1342, w1338, "\t") -> (w1341:string)
                  }
                }
                n1100 = property on="Figure_axis" class="Arr (strict)"("Value"=w1330) -> ()  [unwired: 2 in, 2 out]
                n1101 = property on="data_caption" class="Str"("Value"=w1332) -> ()  [unwired: 2 in, 2 out]
              }
              frame #5 {
                # "SR830 3 out of phase (SR830_3_oop)"
                n1102 = local read "SR830 3 oop"() -> (w1349:bool)
                n1103 = property on="Figure_axis" class="Arr (strict)"() -> ("Value"=w1346:string[])  [unwired: 2 in, 2 out]
                n1104 = property on="data_caption" class="Str"() -> ("Value"=w1348:string)  [unwired: 2 in, 2 out]
                n1105 = case shown="False" w1349 {
                  tunnel: w1348 -> [w1351 w1357]
                  tunnel: [w1351 w1356] -> w1347
                  tunnel: w1346 -> [w1350 w1354]
                  tunnel: [w1350 w1352] -> w1345
                  frame False {
                    # "not measure SR830 3 out of phase signal (SR830_3_oop)"
                  }
                  frame True {
                    w1353 = "SR830_3_oop"
                    # "measure SR830 3 out phase signal (SR830_3_oop)"
                    n1106 = local read "SR830 3 addr"() -> (w1358:u8)
                    n1107 = Number To Decimal String(number=w1358) -> (decimal integer string=w1359:string)  [unwired: 1 in]
                    n1108 = GPIB Clear(3:w1359) -> ()  [unwired: 1 in, 2 out]
                    n1109 = Build Array (concatenate)(w1354, w1353) -> (w1352:string[])
                    n1110 = Concatenate Strings(w1357, w1353, "\t") -> (w1356:string)
                  }
                }
                n1111 = property on="Figure_axis" class="Arr (strict)"("Value"=w1345) -> ()  [unwired: 2 in, 2 out]
                n1112 = property on="data_caption" class="Str"("Value"=w1347) -> ()  [unwired: 2 in, 2 out]
              }
              frame #6 {
                # "SR830 4 in phase (SR830_4_ip)"
                n1113 = local read "SR830 4 ip"() -> (w1364:bool)
                n1114 = property on="Figure_axis" class="Arr (strict)"() -> ("Value"=w1361:string[])  [unwired: 2 in, 2 out]
                n1115 = property on="data_caption" class="Str"() -> ("Value"=w1363:string)  [unwired: 2 in, 2 out]
                n1116 = case shown="False" w1364 {
                  tunnel: w1363 -> [w1366 w1372]
                  tunnel: [w1366 w1371] -> w1362
                  tunnel: w1361 -> [w1365 w1369]
                  tunnel: [w1365 w1367] -> w1360
                  frame False {
                    # "not measure SR830 4 in phase signal (SR830_4_ip)"
                  }
                  frame True {
                    w1368 = "SR830_4_ip"
                    # "measure SR830 4 in phase signal (SR830_4_ip)"
                    n1117 = local read "SR830 4 addr"() -> (w1373:u8)
                    n1118 = Number To Decimal String(number=w1373) -> (decimal integer string=w1374:string)  [unwired: 1 in]
                    n1119 = GPIB Clear(3:w1374) -> ()  [unwired: 1 in, 2 out]
                    n1120 = Build Array (concatenate)(w1369, w1368) -> (w1367:string[])
                    n1121 = Concatenate Strings(w1372, w1368, "\t") -> (w1371:string)
                  }
                }
                n1122 = property on="Figure_axis" class="Arr (strict)"("Value"=w1360) -> ()  [unwired: 2 in, 2 out]
                n1123 = property on="data_caption" class="Str"("Value"=w1362) -> ()  [unwired: 2 in, 2 out]
              }
              frame #7 {
                # "SR830 4 out of phase (SR830_4_oop)"
                n1124 = local read "SR830 4 oop"() -> (w1379:bool)
                n1125 = property on="Figure_axis" class="Arr (strict)"() -> ("Value"=w1376:string[])  [unwired: 2 in, 2 out]
                n1126 = property on="data_caption" class="Str"() -> ("Value"=w1378:string)  [unwired: 2 in, 2 out]
                n1127 = case shown="False" w1379 {
                  tunnel: w1378 -> [w1381 w1387]
                  tunnel: [w1381 w1386] -> w1377
                  tunnel: w1376 -> [w1380 w1384]
                  tunnel: [w1380 w1382] -> w1375
                  frame False {
                    # "not measure SR830 4 out of phase signal (SR830_4_oop)"
                  }
                  frame True {
                    w1383 = "SR830_4_oop"
                    # "measure SR830 4 out of phase signal (SR830_4_oop)"
                    n1128 = local read "SR830 4 addr"() -> (w1388:u8)
                    n1129 = Number To Decimal String(number=w1388) -> (decimal integer string=w1389:string)  [unwired: 1 in]
                    n1130 = GPIB Clear(3:w1389) -> ()  [unwired: 1 in, 2 out]
                    n1131 = Build Array (concatenate)(w1384, w1383) -> (w1382:string[])
                    n1132 = Concatenate Strings(w1387, w1383, "\t") -> (w1386:string)
                  }
                }
                n1133 = property on="Figure_axis" class="Arr (strict)"("Value"=w1375) -> ()  [unwired: 2 in, 2 out]
                n1134 = property on="data_caption" class="Str"("Value"=w1377) -> ()  [unwired: 2 in, 2 out]
              }
              frame #8 {
                # "2400 1 voltage measure (2400_1_v)"
                n1135 = local read "2400 1 meas v"() -> (w1394:bool)
                n1136 = property on="Figure_axis" class="Arr (strict)"() -> ("Value"=w1391:string[])  [unwired: 2 in, 2 out]
                n1137 = property on="data_caption" class="Str"() -> ("Value"=w1393:string)  [unwired: 2 in, 2 out]
                n1138 = case shown="False" w1394 {
                  tunnel: w1393 -> [w1396 w1402]
                  tunnel: [w1396 w1401] -> w1392
                  tunnel: w1391 -> [w1395 w1399]
                  tunnel: [w1395 w1397] -> w1390
                  frame False {
                    # "not measure 2400 1 voltage (2400_1_v)"
                  }
                  frame True {
                    w1398 = "2400_1_v"
                    # "measure 2400 1 voltage (2400_1_v)"
                    n1139 = local read "2400 1 addr"() -> (w1403:u8)
                    n1140 = Number To Decimal String(number=w1403) -> (decimal integer string=w1404:string)  [unwired: 1 in]
                    n1141 = GPIB Clear(3:w1404) -> ()  [unwired: 1 in, 2 out]
                    n1142 = Build Array (concatenate)(w1399, w1398) -> (w1397:string[])
                    n1143 = Concatenate Strings(w1402, w1398, "\t") -> (w1401:string)
                  }
                }
                n1144 = property on="Figure_axis" class="Arr (strict)"("Value"=w1390) -> ()  [unwired: 2 in, 2 out]
                n1145 = property on="data_caption" class="Str"("Value"=w1392) -> ()  [unwired: 2 in, 2 out]
              }
              frame #9 {
                # "2400 1 current measure (2400_1_i)"
                n1146 = local read "2400 1 meas i"() -> (w1409:bool)
                n1147 = property on="Figure_axis" class="Arr (strict)"() -> ("Value"=w1406:string[])  [unwired: 2 in, 2 out]
                n1148 = property on="data_caption" class="Str"() -> ("Value"=w1408:string)  [unwired: 2 in, 2 out]
                n1149 = case shown="False" w1409 {
                  tunnel: w1408 -> [w1411 w1417]
                  tunnel: [w1411 w1416] -> w1407
                  tunnel: w1406 -> [w1410 w1414]
                  tunnel: [w1410 w1412] -> w1405
                  frame False {
                    # "not measure 2400 1 current (2400_1_i)"
                  }
                  frame True {
                    w1413 = "2400_1_i"
                    # "measure 2400 1 current (2400_1_i)"
                    n1150 = local read "2400 1 addr"() -> (w1418:u8)
                    n1151 = Number To Decimal String(number=w1418) -> (decimal integer string=w1419:string)  [unwired: 1 in]
                    n1152 = GPIB Clear(3:w1419) -> ()  [unwired: 1 in, 2 out]
                    n1153 = Build Array (concatenate)(w1414, w1413) -> (w1412:string[])
                    n1154 = Concatenate Strings(w1417, w1413, "\t") -> (w1416:string)
                  }
                }
                n1155 = property on="Figure_axis" class="Arr (strict)"("Value"=w1405) -> ()  [unwired: 2 in, 2 out]
                n1156 = property on="data_caption" class="Str"("Value"=w1407) -> ()  [unwired: 2 in, 2 out]
              }
              frame #10 {
                # "2400 2 voltage measure (2400_2_v)"
                n1157 = local read "2400 2 meas v"() -> (w1424:bool)
                n1158 = property on="Figure_axis" class="Arr (strict)"() -> ("Value"=w1421:string[])  [unwired: 2 in, 2 out]
                n1159 = property on="data_caption" class="Str"() -> ("Value"=w1423:string)  [unwired: 2 in, 2 out]
                n1160 = case shown="False" w1424 {
                  tunnel: w1423 -> [w1426 w1432]
                  tunnel: [w1426 w1431] -> w1422
                  tunnel: w1421 -> [w1425 w1429]
                  tunnel: [w1425 w1427] -> w1420
                  frame False {
                    # "not measure 2400 2 voltage (2400_2_v)"
                  }
                  frame True {
                    w1428 = "2400_2_v"
                    # "measure 2400 2 voltage (2400_2_v)"
                    n1161 = local read "2400 2 addr"() -> (w1433:u8)
                    n1162 = Number To Decimal String(number=w1433) -> (decimal integer string=w1434:string)  [unwired: 1 in]
                    n1163 = GPIB Clear(3:w1434) -> ()  [unwired: 1 in, 2 out]
                    n1164 = Build Array (concatenate)(w1429, w1428) -> (w1427:string[])
                    n1165 = Concatenate Strings(w1432, w1428, "\t") -> (w1431:string)
                  }
                }
                n1166 = property on="Figure_axis" class="Arr (strict)"("Value"=w1420) -> ()  [unwired: 2 in, 2 out]
                n1167 = property on="data_caption" class="Str"("Value"=w1422) -> ()  [unwired: 2 in, 2 out]
              }
              frame #11 {
                # "2400 2 current measure (2400_2_i)"
                n1168 = local read "2400 2 meas i"() -> (w1439:bool)
                n1169 = property on="Figure_axis" class="Arr (strict)"() -> ("Value"=w1436:string[])  [unwired: 2 in, 2 out]
                n1170 = property on="data_caption" class="Str"() -> ("Value"=w1438:string)  [unwired: 2 in, 2 out]
                n1171 = case shown="False" w1439 {
                  tunnel: w1438 -> [w1441 w1447]
                  tunnel: [w1441 w1446] -> w1437
                  tunnel: w1436 -> [w1440 w1444]
                  tunnel: [w1440 w1442] -> w1435
                  frame False {
                    # "not measure 2400 2 current (2400_2_i)"
                  }
                  frame True {
                    w1443 = "2400_2_i"
                    # "measure 2400 2 current (2400_2_i)"
                    n1172 = local read "2400 2 addr"() -> (w1448:u8)
                    n1173 = Number To Decimal String(number=w1448) -> (decimal integer string=w1449:string)  [unwired: 1 in]
                    n1174 = GPIB Clear(3:w1449) -> ()  [unwired: 1 in, 2 out]
                    n1175 = Build Array (concatenate)(w1444, w1443) -> (w1442:string[])
                    n1176 = Concatenate Strings(w1447, w1443, "\t") -> (w1446:string)
                  }
                }
                n1177 = property on="Figure_axis" class="Arr (strict)"("Value"=w1435) -> ()  [unwired: 2 in, 2 out]
                n1178 = property on="data_caption" class="Str"("Value"=w1437) -> ()  [unwired: 2 in, 2 out]
              }
              frame #12 {
                # "2400 3 voltage measure (2400_3_v)"
                n1179 = local read "2400 3 meas v"() -> (w1454:bool)
                n1180 = property on="Figure_axis" class="Arr (strict)"() -> ("Value"=w1451:string[])  [unwired: 2 in, 2 out]
                n1181 = property on="data_caption" class="Str"() -> ("Value"=w1453:string)  [unwired: 2 in, 2 out]
                n1182 = case shown="False" w1454 {
                  tunnel: w1453 -> [w1456 w1462]
                  tunnel: [w1456 w1461] -> w1452
                  tunnel: w1451 -> [w1455 w1459]
                  tunnel: [w1455 w1457] -> w1450
                  frame False {
                    # "not measure 2400 3 voltage (2400_3_v)"
                  }
                  frame True {
                    w1458 = "2400_3_v"
                    # "measure 2400 3 voltage (2400_3_v)"
                    n1183 = local read "2400 3 addr"() -> (w1463:u8)
                    n1184 = Number To Decimal String(number=w1463) -> (decimal integer string=w1464:string)  [unwired: 1 in]
                    n1185 = GPIB Clear(3:w1464) -> ()  [unwired: 1 in, 2 out]
                    n1186 = Build Array (concatenate)(w1459, w1458) -> (w1457:string[])
                    n1187 = Concatenate Strings(w1462, w1458, "\t") -> (w1461:string)
                  }
                }
                n1188 = property on="Figure_axis" class="Arr (strict)"("Value"=w1450) -> ()  [unwired: 2 in, 2 out]
                n1189 = property on="data_caption" class="Str"("Value"=w1452) -> ()  [unwired: 2 in, 2 out]
              }
              frame #13 {
                # "2400 3 current measure (2400_3_i)"
                n1190 = local read "2400 3 meas i"() -> (w1469:bool)
                n1191 = property on="Figure_axis" class="Arr (strict)"() -> ("Value"=w1466:string[])  [unwired: 2 in, 2 out]
                n1192 = property on="data_caption" class="Str"() -> ("Value"=w1468:string)  [unwired: 2 in, 2 out]
                n1193 = case shown="True" w1469 {
                  tunnel: w1468 -> [w1471 w1477]
                  tunnel: [w1471 w1476] -> w1467
                  tunnel: w1466 -> [w1470 w1474]
                  tunnel: [w1470 w1472] -> w1465
                  frame False {
                    # "not measure 2400 3 current (2400_3_i)"
                  }
                  frame True {
                    w1473 = "2400_3_i"
                    # "measure 2400 3 current (2400_3_i)"
                    n1194 = local read "2400 3 addr"() -> (w1478:u8)
                    n1195 = Number To Decimal String(number=w1478) -> (decimal integer string=w1479:string)  [unwired: 1 in]
                    n1196 = GPIB Clear(3:w1479) -> ()  [unwired: 1 in, 2 out]
